vi "PrácticaSalidaContinua.vi"() -> ()   [LabVIEW 2016]
uses:
  <vilib>/DAQmx/read.llb/DAQmx Read (Analog DBL 1Chan 1Samp).vi
  <vilib>/DAQmx/write.llb/DAQmx Write (Analog 1D DBL NChan 1Samp).vi
  <vilib>/DAQmx/create/channels.llb/DAQmx Create Channel (AI-Voltage-Basic).vi
  <vilib>/DAQmx/configure/timing.llb/DAQmx Timing (Sample Clock).vi
  <vilib>/DAQmx/create/channels.llb/DAQmx Create Channel (AO-Voltage-Basic).vi
  <vilib>/DAQmx/miscellaneous.llb/DAQmx Fill In Error Info.vi
panel:
  in  "señal":path
  in  "f":path
  in  "integral":path
  out "Derivada":dbl(graph)
  out "Integral":dbl(graph)
  out "Señal":dbl(graph)
  in  "Stop Button":bool
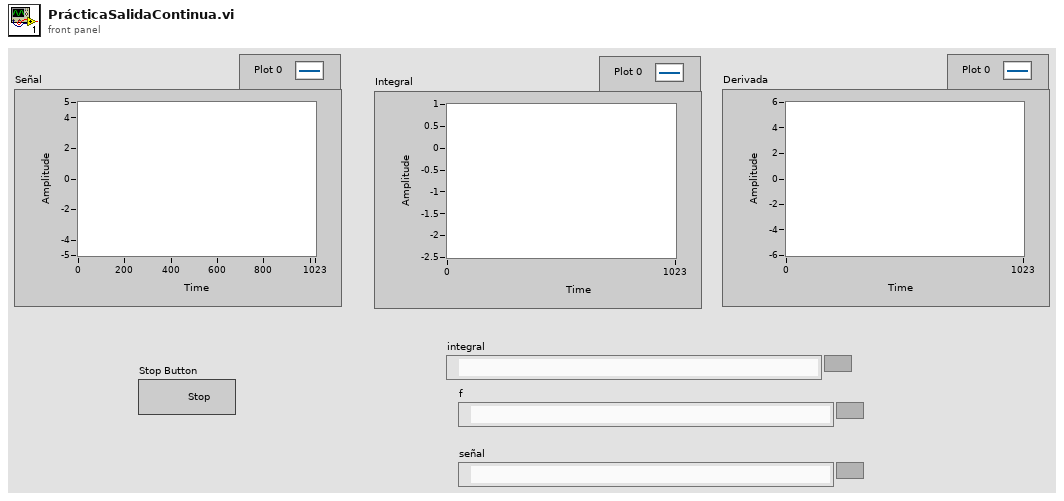
[diagram p1: front panel]
types:
  T1 = enum16{"open", "replace", "create", "open or create", "replace or create", "replace or create with confirmation"}
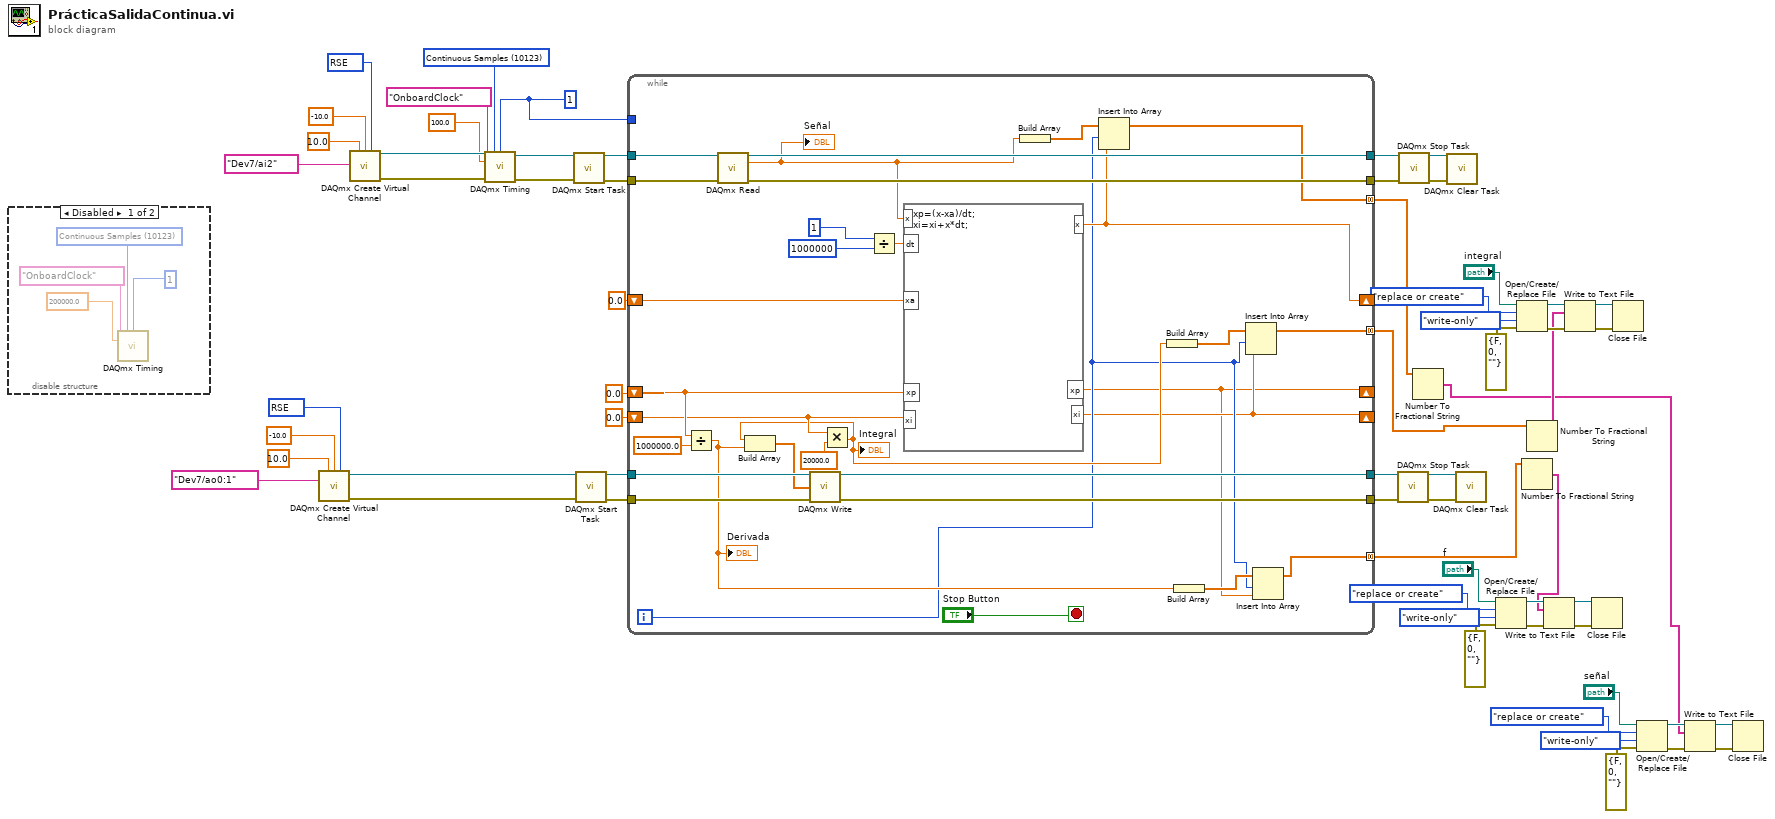
[diagram p0: block diagram]
diagram:
  w40 = 10083 items=["Default"=-1, "RSE"=10083, "Differential"=10106, "Pseudodifferential"=12529] ("output terminal configuration")
  w50 = 1 ("samples per channel")
  w56 = 10123 items=["Finite Samples"=10178, "Continuous Samples"=10123, "Hardware Timed Single Point"=12522] ("sample mode")
  w61 = 10083 items=["Default"=-1, "RSE"=10083, "NRSE"=10078, "Differential"=10106, "Pseudodifferential"=12529] ("input terminal configuration")
  n1 = disable-structure shown="Disabled" {
    frame Disabled {
      w65 = 10123 items=["Finite Samples"=10178, "Continuous Samples"=10123, "Hardware Timed Single Point"=12522] ("sample mode")
      n2 = call-poly <vilib>:"DAQmx Timing.vi"("sample mode"=w65, "samples per channel"=1, "rate"=200000.0, "source"=tag "OnboardClock") -> ()  [unwired: 10 in, 2 out]
    }
    frame Enabled {
    }
  }
  n3 = call-poly <vilib>:"DAQmx Create Virtual Channel.vi"("maximum value"=10.0, "minimum value"=-10.0, "output terminal configuration"=w40, "physical channels"=tag "Dev7/ao0:1") -> ("task out"=w32:refnum<k21>, "error out"=w31:errorcluster)  [unwired: 10 in]
  n4 = call-poly <vilib>:"DAQmx Create Virtual Channel.vi"("maximum value"=10.0, "minimum value"=-10.0, "input terminal configuration"=w61, "physical channels"=tag "Dev7/ai2") -> ("task out"=w58:refnum<k21>, "error out"=w59:errorcluster)  [unwired: 10 in]
  n5 = call-poly <vilib>:"DAQmx Timing.vi"("task/channels in"=w58, "sample mode"=w56, "samples per channel"=w50, "rate"=100.0, "source"=tag "OnboardClock", "error in"=w59) -> ("task out"=w53:refnum<k21>, "error out"=w54:errorcluster)  [unwired: 8 in]
  n6 = call <vilib>:"DAQmx Start Task.vi"("task/channels in"=w53, "error in"=w54) -> ("task out"=w52:refnum<k21>, "error out"=w51:errorcluster)  [unwired: 12 in]
  n7 = call <vilib>:"DAQmx Start Task.vi"("task/channels in"=w32, "error in"=w31) -> ("task out"=w38:refnum<k21>, "error out"=w37:errorcluster)  [unwired: 12 in]
  n8 = while {
    tunnel: w50 -> [_]
    shift-right: [w70] -> _
    shift-left: 0.0 -> [w84]
    shift-right: [w71] -> _
    shift-left: 0.0 -> [w83]
    shift-right: [w77] -> _
    shift-left: 0.0 -> [w91]
    tunnel: w38 -> [w90]
    tunnel: w37 -> [w89]
    tunnel: [w88] -> w34
    tunnel: [w87] -> w33
    tunnel: w52 -> [w98]
    tunnel: [w96] -> w49
    tunnel: w51 -> [w97]
    tunnel: [w95] -> w48
    tunnel: [w78] -> w4 mode=concatenating
    tunnel: [w69] -> w2 mode=concatenating
    tunnel: [w68] -> w1 mode=concatenating
    i -> [w72]
    stop <- "Stop Button" stop-if-true
    n9 = Divide(x=w84, y=1000000.0) -> (x/y=w73:dbl)
    "Derivada" <- w73
    n10 = call-poly <vilib>:"DAQmx Read.vi"("task/channels in"=w98, "error in"=w97) -> ("task out"=w96:refnum<k21>, "data"=w80:dbl, "error out"=w95:errorcluster)  [unwired: 11 in]
    "Señal" <- w80
    n11 = Multiply(x=w83, y=20000.0) -> (x*y=w75:dbl)
    "Integral" <- w75
    n12 = Build Array(w75, w73) -> (w81:dbl[])
    n13 = call-poly <vilib>:"DAQmx Write.vi"("task/channels in"=w90, "data"=w81, "error in"=w89) -> ("task out"=w88:refnum<k21>, "error out"=w87:errorcluster)  [unwired: 10 in, 1 out]
    n14 = Divide(x=u32 1 ("milliseconds to wait"), y=u32 1000000) -> (x/y=w93:dbl)
    n15 = formula code="xp=(x-xa)/dt;\nxi=xi+x*dt;"("x"=w80, "xp"=w84, "dt"=w93, "xi"=w83, "xa"=w91) -> ("x"=w77:dbl, "xp"=w70:dbl, "xi"=w71:dbl)
    n16 = Build Array(w80) -> (w79:dbl[])
    n17 = Insert Into Array(array=w79, index=w72, new element=w77) -> (w78:dbl[])
    n18 = Build Array(w75) -> (w76:dbl[])
    n19 = Build Array(w73) -> (w74:dbl[])
    n20 = Insert Into Array(array=w76, index=w72, new element=w71) -> (w69:dbl[])
    n21 = Insert Into Array(array=w74, index=w72, new element=w70) -> (w68:dbl[])
  }
  n22 = call <vilib>:"DAQmx Stop Task.vi"("task/channels in"=w34, "error in"=w33) -> ("task out"=w36:refnum<k21>, "error out"=w35:errorcluster)  [unwired: 12 in]
  n23 = call <vilib>:"DAQmx Stop Task.vi"("task/channels in"=w49, "error in"=w48) -> ("task out"=w47:refnum<k21>, "error out"=w46:errorcluster)  [unwired: 12 in]
  n24 = Number To Fractional String(number=w4) -> (F-format string=w3:string[])  [unwired: 3 in]
  n25 = call <vilib>:"DAQmx Clear Task.vi"("task in"=w47, "error in"=w46) -> ()  [unwired: 13 in, 1 out]
  n26 = call <vilib>:"DAQmx Clear Task.vi"("task in"=w36, "error in"=w35) -> ()  [unwired: 13 in, 1 out]
  n27 = Open/Create/Replace File(file path (use dialog)="f", error in=errorcluster {"status"=FALSE, "code"=0, "source"=""}, operation (0:open)=T1."replace or create", access (0:read/write)=enum16{"read/write", "read-only", "write-only"}."write-only") -> (refnum out=w17:refnum<file>, error out=w18:errorcluster)  [unwired: 2 in, 1 out]
  n28 = Open/Create/Replace File(file path (use dialog)="integral", error in=errorcluster {"status"=FALSE, "code"=0, "source"=""}, operation (0:open)=T1."replace or create", access (0:read/write)=enum16{"read/write", "read-only", "write-only"}."write-only") -> (refnum out=w25:refnum<file>, error out=w26:errorcluster)  [unwired: 2 in, 1 out]
  n29 = Number To Fractional String(number=w1) -> (F-format string=w5:string[])  [unwired: 3 in]
  n30 = Number To Fractional String(number=w2) -> (F-format string=w6:string[])  [unwired: 3 in]
  n31 = Write to Text File(file (use dialog)=w17, text=w5, error in=w18) -> (refnum out=w15:refnum<file>, error out=w16:errorcluster)  [unwired: 1 in, 1 out]
  n32 = Write to Text File(file (use dialog)=w25, text=w6, error in=w26) -> (refnum out=w23:refnum<file>, error out=w24:errorcluster)  [unwired: 1 in, 1 out]
  n33 = Close File(refnum=w15, error in=w16) -> ()  [unwired: 2 out]
  n34 = Close File(refnum=w23, error in=w24) -> ()  [unwired: 2 out]
  n35 = Open/Create/Replace File(file path (use dialog)="señal", error in=errorcluster {"status"=FALSE, "code"=0, "source"=""}, operation (0:open)=T1."replace or create", access (0:read/write)=enum16{"read/write", "read-only", "write-only"}."write-only") -> (refnum out=w9:refnum<file>, error out=w10:errorcluster)  [unwired: 2 in, 1 out]
  n36 = Write to Text File(file (use dialog)=w9, text=w3, error in=w10) -> (refnum out=w7:refnum<file>, error out=w8:errorcluster)  [unwired: 1 in, 1 out]
  n37 = Close File(refnum=w7, error in=w8) -> ()  [unwired: 2 out]
